vi "Caption Test.vi"() -> ()   [LabVIEW 2019]
uses:
  uiControlsMgr.lvclass
panel:
  out "0007":bool caption="MAIS LONGO"
  out "0006":bool caption="PARTIDA"
  out "0008":bool caption="REPETE"
  in  "0005":dbl(slide) caption="HABILIDADE" scale=0.0..10.0
  in  "0004":bool caption="Amarelo"
  in  "0003":bool caption="Verde"
  in  "0002":bool caption="Azul"
  in  "0001":bool caption="Vermelho"
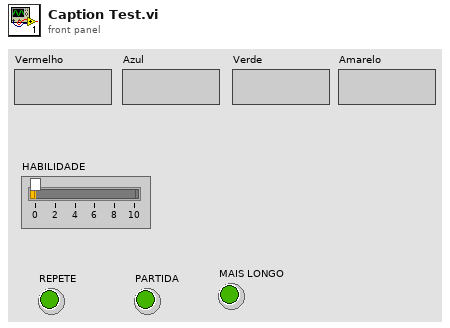
[diagram p1: front panel]
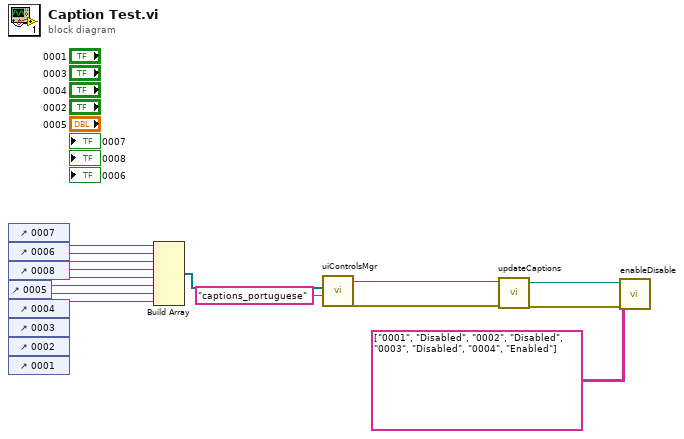
[diagram p0: block diagram]
diagram:
  n1 = control-ref of="0007"() -> (w13:refnum<vi>)
  n2 = control-ref of="0006"() -> (w12:refnum<vi>)
  n3 = control-ref of="0008"() -> (w11:refnum<vi>)
  n4 = control-ref of="0005"() -> (w10:refnum<vi>)
  n5 = control-ref of="0004"() -> (w9:refnum<vi>)
  n6 = control-ref of="0003"() -> (w8:refnum<vi>)
  n7 = control-ref of="0002"() -> (w7:refnum<vi>)
  n8 = control-ref of="0001"() -> (w6:refnum<vi>)
  n9 = Build Array(w13, w12, w11, w10, w9, w8, w7, w6) -> (w5:refnum<vi>[])
  n10 = call "uiControlsMgr.vi"("Captions File"="captions_portuguese", "UI Refnums"=w5) -> ("error out"=w14:errorcluster, "uiControlsMgr out"=w15:refnum<class "uiControlsMgr.lvclass">)  [unwired: 8 in]
  n11 = call "updateCaptions.vi"("error in (no error)"=w14, "uiControlsMgr in"=w15) -> ("error out"=w2:errorcluster, "uiControlsMgr out"=w3:refnum<class "uiControlsMgr.lvclass">)  [unwired: 8 in]
  n12 = call "enableDisable.vi"("error in (no error)"=w2, "Controls - Status"=string[][] [["0001", "Disabled"], ["0002", "Disabled"], ["0003", "Disabled"], ["0004", "Enabled"]], "uiControlsMgr in"=w3) -> ()  [unwired: 7 in, 2 out]
